vi "Test Discovery Beacon.vi"() -> ()   [LabVIEW 2020]
uses:
  Source/epl-network.lvlib
panel:
  in  "stop":bool
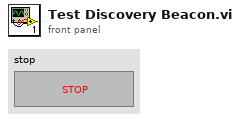
[diagram p1: front panel]
types:
  T1 = typedef "epl-network.lvlib/IPEndPoint.ctl" = cluster{"address":string, "port":i32}
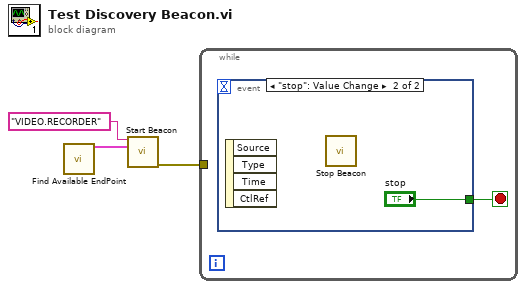
[diagram p0: block diagram]
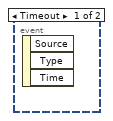
[diagram p2: hidden frame]
diagram:
  n1 = call "Find Available EndPoint.vi"() -> ("IPEndPoint"=w3:T1)  [unwired: 14 in, 1 out]
  n2 = call "Start Beacon.vi"("name"="VIDEO.RECORDER", "TCP Server EndPoint"=w3) -> ("error out"=w1:errorcluster)  [unwired: 13 in]
  n3 = while {
    tunnel: w1 -> [_]
    stop <- w4 stop-if-true
    n4 = event shown="[1] \"stop\": Value Change" {
      selector: _ -> [_ _]
      dyn-events: _ -> [_ _]
      timeout: _ -> [_ _]
      tunnel: [_ "stop"] -> w4
      event Timeout {
        n5 = event-data() -> ()  [unwired: 1 in, 3 out]
      }
      event "stop": Value Change {
        n6 = event-data() -> ()  [unwired: 1 in, 4 out]
        n7 = call "Stop Beacon.vi"() -> ()  [unwired: 12 in]
      }
    }
  }
